vi "ASIA Reserve Pump.vi"(8 "error in (no error)":errorcluster, 11 "ASIA Pump #":i32) -> (0 "error out":errorcluster, 3 "ASIA Pump #":i32)   [LabVIEW 2018, in "ASIA Pump.lvlib"]
uses:
  ASIA Pump.lvlib
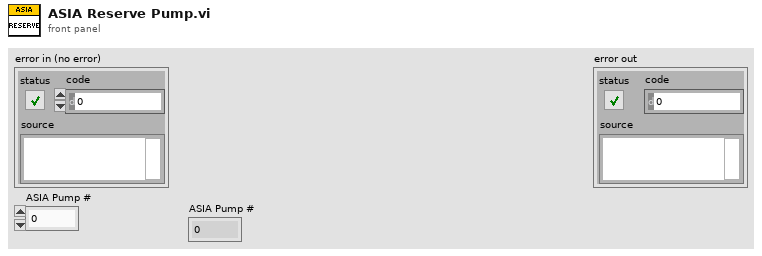
[diagram p1: front panel]
types:
  T1 = cluster{"Busy":bool, "PumpCnt":dbl, "RemoteEntered":bool, "OverpressureSet":bool}[]
  T2 = cluster{"Busy":bool, "PumpCnt":dbl, "RemoteEntered":bool, "OverpressureSet":bool}
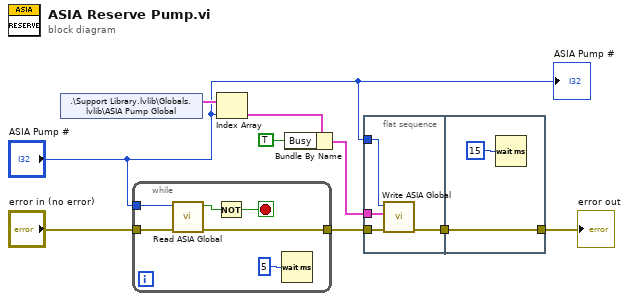
[diagram p0: block diagram]
diagram:
  n1 = shared-variable ".\\Support Library.lvlib\\Globals.lvlib\\ASIA Pump Global"() -> (w3:T1)  [unwired: 1 in, 1 out]
  n2 = while {
    tunnel: "ASIA Pump #" -> [w15]
    tunnel: [w12] -> w9
    tunnel: "error in (no error)" -> [w11]
    stop <- w13 stop-if-true
    n3 = call "Read ASIA Global.vi"("error in (no error)"=w11, "Pump Number"=w15) -> ("error out"=w12:errorcluster, "Busy"=w14:bool)  [unwired: 8 in]
    n4 = Not(x=w14) -> (.not. x?=w13:bool)
    n5 = Wait (ms)(milliseconds to wait=u32 5) -> ()  [unwired: 1 out]
  }
  n6 = Index Array(array=w3, index="ASIA Pump #") -> (element=w4:T2)
  n7 = Bundle By Name(cluster=w4, "Busy"=TRUE) -> (w5:T2)
  n8 = flat-sequence {
    tunnel: w9 -> [w19]
    tunnel: w5 -> [w17]
    tunnel: "ASIA Pump #" -> [w16]
    tunnel: [w18] -> w1
    tunnel: [w21] -> w7
    tunnel: w1 -> [w21]
    frame #0 {
      n9 = call "Write ASIA Global.vi"("error in (no error)"=w19, "ASIA Global"=w17, "Pump Number"=w16) -> ("error out"=w18:errorcluster)  [unwired: 7 in, 1 out]
    }
    frame #1 {
      n10 = Wait (ms)(milliseconds to wait=u32 15) -> ()  [unwired: 1 out]
    }
  }
  "error out" <- w7
  "ASIA Pump #" <- "ASIA Pump #"
